vi "Reset.vi"(8 "error in (no error)":errorcluster, 10 "gRPCid":T2, 11 "ctet_mux in":T1) -> (0 "error out":errorcluster, 3 "ctet_mux out":T1)   [LabVIEW 2019, in "ctet_mux_User Library.lvlib"]
uses:
  ctet_mux_User Library.lvlib
  Servers/ctet_mux/gRPC lvSupport/Server API/typeDefs/grpcId.ctl
  Types/ctet_mux.ctl
  Servers/ctet_mux/ctet_mux Class/RPC Messages/measurementservice_MUXResetResponse/measurementservice_MUXResetResponse_Data.ctl
  Servers/ctet_mux/ctet_mux Class/RPC Messages/measurementservice_ErrorOut/measurementservice_ErrorOut_Data.ctl
  Types/Switch Action.ctl
  Servers/ctet_mux/ctet_mux Class/ctet_mux.lvclass
  Servers/ctet_mux/gRPC lvSupport/gprc-lvsupport.lvlib
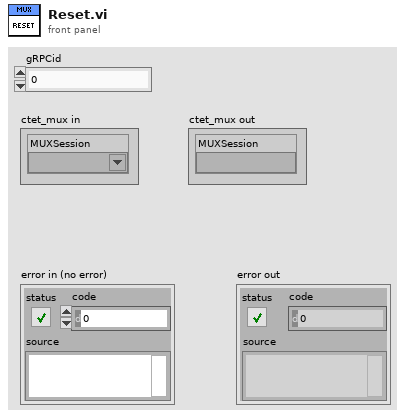
[diagram p1: front panel]
types:
  T1 = typedef "ctet_mux_User Library.lvlib/ctet_mux.ctl" = cluster{"MUXSession":refnum<k15>}
  T2 = typedef "ctet_mux.lvlib/gprc-lvsupport.lvlib/grpcId.ctl" = u64
  T3 = typedef "ctet_mux_User Library.lvlib/Switch Action.ctl" = enum16{"Get Switch State", "Initialize", "Connect Channel", "Open Channel", "Close Relay", "Open Relay", "Disconnect/Open All"}
  T4 = typedef "ctet_mux.lvlib/ctet_mux.lvclass/measurementservice_ErrorOut_Data.ctl" = cluster{"errCode":i64, "errMessage":string}
  T5 = typedef "ctet_mux.lvlib/ctet_mux.lvclass/measurementservice_MUXResetResponse_Data.ctl" = cluster{"error":T4}
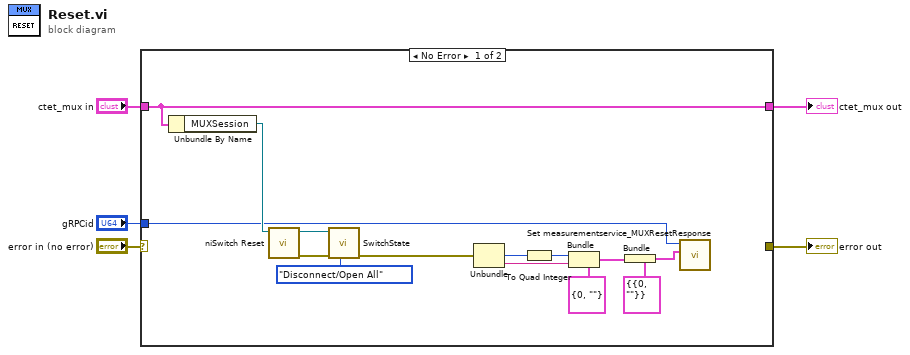
[diagram p0: block diagram]
diagram:
  n1 = case shown="No Error" "error in (no error)" {
    selector: "error in (no error)" -> [_ w21]
    tunnel: [_ w21] -> w5
    tunnel: "gRPCid" -> [w14 _]
    tunnel: "ctet_mux in" -> [w15 w20]
    tunnel: [w15 w20] -> w1
    frame No Error {
      n2 = Unbundle By Name(w15) -> ("MUXSession"=w16:refnum<k15>)
      n3 = call <instrlib>:"niSwitch Reset.vi"("instrument handle"=w16) -> ("error out"=w9:errorcluster, "instrument handle out"=w7:refnum<k15>)  [unwired: 9 in]
      n4 = call "SwitchState.vi"("Switch Action"=Switch_Action."Disconnect/Open All", "error in (no error)"=w9, "Switch Session"=w7) -> ("error out"=w8:errorcluster)  [unwired: 6 in, 2 out]
      n5 = Unbundle(w8) -> ("code"=w18:i32, "source"=w19:string)  [unwired: 1 out]
      n6 = To Quad Integer(1:w18) -> (0:w17:i64)
      n7 = Bundle(cluster=T4 {"errCode"=0, "errMessage"=""} ("error"), "errCode"=w17, "errMessage"=w19) -> (w10:T4)
      n8 = Bundle(cluster=T5 {"error"={"errCode"=0, "errMessage"=""}} ("measurementservice_MUXResetResponse_Data"), "error"=w10) -> (w13:T5)
      n9 = call "Set measurementservice_MUXResetResponse.vi"("Message Data"=w13, "gRPCid"=w14) -> ()  [unwired: 9 in, 1 out]
    }
    frame Error {
    }
  }
  "error out" <- w5
  "ctet_mux out" <- w1
